vi "Lipgap Algo.vi"(8 "error in":errorcluster, 11 "Image In":T1) -> (0 "error out":errorcluster, 1 "Edge CG":cluster{"X":sgl, "Y":sgl}[](array[cluster]) {"Y" format="%.2f"; "X" format="%.2f"}, 2 "Image":T1(plugin-control), 3 "Image Out":T1(plugin-control), 4 "Edge points Height":cluster{"X":sgl, "Y":sgl}[](array[cluster]))   [LabVIEW 2015]
uses:
  FrameworkOverrides/Algorithm.lvclass
  <vilib>/vision/Image Controls.llb/IMAQ Image.ctl
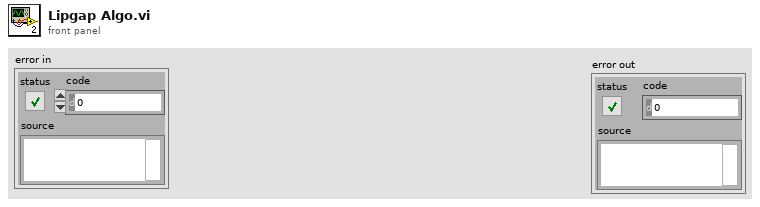
[diagram p1: front panel]
types:
  T1 = typedef "IMAQ Image.ctl" = refnum<image>
  T2 = cluster{"Lower thresh":sgl, "Upper thresh":sgl, "Xoffset":sgl, "Y offset":sgl}
  T3 = cluster{"Start x offset":sgl, "End x offset":sgl, "Start y offset":sgl, "End y offset":sgl, "Carrier offset":sgl, "Height":sgl, "X left":sgl, "X right":sgl, "Angle":sgl}
  T4 = typedef "ROI Descriptor" = cluster{"Global Rectangle":i32[], "Contours":cluster{"ID":enum32{"External", "Internal"}, "Type":u32, "Coordinates":i32[]}[]}
  T5 = cluster{"Left":i32, "Top":i32, "Right":i32, "Bottom":i32}
  T6 = typedef "Edge New.ctl" = cluster{"Location (Pixel)":cluster{"X":sgl, "Y":sgl}, "Location (Real-World)":cluster{"X":sgl, "Y":sgl}, "Distance (Pixel)":dbl, "Distance (Real-World)":dbl, "Strength":dbl, "Noise":dbl, "Rising?":bool}
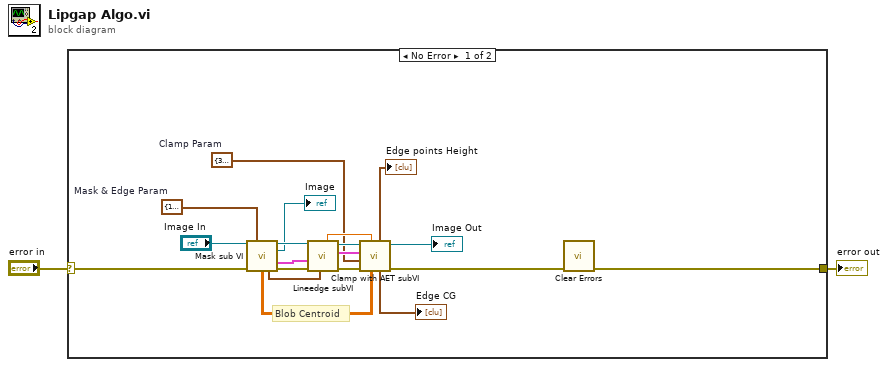
[diagram p0: block diagram]
diagram:
  n1 = case shown="No Error" "error in" {
    selector: "error in" -> [w9 _]
    tunnel: [w10 _] -> w1
    frame No Error {
      w3 = T2 {"Lower thresh"=100.0, "Upper thresh"=255.0, "Xoffset"=30.0, "Y offset"=60.0}  # Mask & Edge Param
      w4 = T3 {"Start x offset"=30.0, "End x offset"=50.0, "Start y offset"=20.0, "End y offset"=25.0, "Carrier offset"=170.0, "Height"=150.0, "X left"=200.0, "X right"=850.0, "Angle"=0.0}  # Clamp Param
      # "Blob Centroid"
      n2 = call "Mask sub VI.vi"("Image In"="Image In", "Mask&Edge ROI param"=w3, "error out"=w9) -> ("Gray Level Image out"=w13:T1, "Binary Image out"=→"Image":T1, "ROI Descriptor"=w19:T4, "Centroid of blob"=w12:dbl[][], "Rectangle for overlay"=w11:T5, "error out"=w18:errorcluster)  [unwired: 7 in]
      n3 = call "Lineedge subVI.vi"("Rectangle for overlay"=w11, "error in (no error)"=w18, "ROI Descriptor"=w19, "Gray Level Image"=w13) -> ("error out"=w17:errorcluster, "All straight Edges"=w16:cluster{"Edge Information":T6[]}[], "Gray level Image"=w14:T1, "Angle (Pixel)"=w15:dbl)  [unwired: 4 in]
      n4 = call "Clamp with AET subVI.vi"("Centroid of blob"=w12, "Angle (Pixel)"=w15, "error in (no error)"=w17, "Clamp param"=w4, "All straight Edges"=w16, "Gray Level Image"=w14) -> ("error out"=w20:errorcluster, "Image Out"=→"Image Out":T1, "Edge points CG"=→"Edge CG":cluster{"X":sgl, "Y":sgl}[], "Edge points Height"=→"Edge points Height":cluster{"X":sgl, "Y":sgl}[])  [unwired: 1 in, 1 out]
      n5 = call <vilib>:"Clear Errors.vi"("error in (no error)"=w20) -> ("error out"=w10:errorcluster)  [unwired: 5 in, 1 out]
    }
    frame Error {
    }
  }
  "error out" <- w1
